vi "Opcode at X.vi"(9 "X Position":enum16{"First", "Second", "Third", "Fourth"}(ring), 11 "Opcode":u16 format="%04x") -> (2 "Opcode at X Position (U8)":u8 format="%02x")   [LabVIEW 2018]
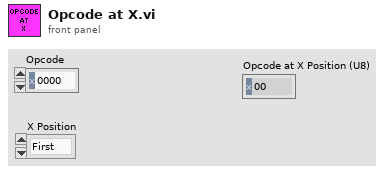
[diagram p1: front panel]
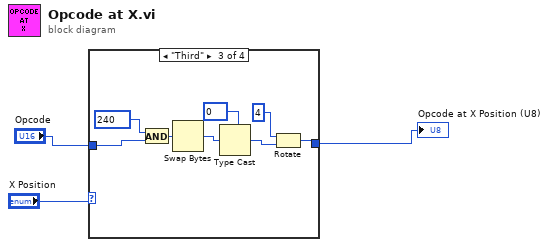
[diagram p0: block diagram]
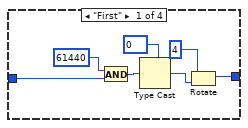
[diagram p2: hidden frame]
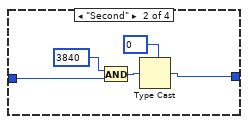
[diagram p3: hidden frame]
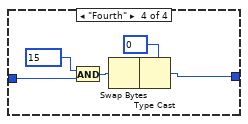
[diagram p4: hidden frame]
diagram:
  n1 = case shown="\"Third\"" "X Position" {
    tunnel: "Opcode" -> [w7 w12 w20 w26]
    tunnel: [w6 w11 w18 w25] -> w1
    frame "First" {
      n2 = And(x=u16 61440 ("y"), y=w7) -> (x .and. y?=w9:u16)
      n3 = Type Cast(type=u8 0, x=w9) -> (*(type *) &x=w5:u8)
      n4 = Rotate(1:w5, 2:u8 4 ("x")) -> (0:w6:u8)
    }
    frame "Second" {
      n5 = And(x=u16 3840 ("y"), y=w12) -> (x .and. y?=w14:u16)
      n6 = Type Cast(type=u8 0, x=w14) -> (*(type *) &x=w11:u8)
    }
    frame "Third" {
      n7 = And(x=u16 240 ("y"), y=w20) -> (x .and. y?=w22:u16)
      n8 = Swap Bytes(anything=w22) -> (byte swapped=w19:u16)
      n9 = Type Cast(type=u8 0, x=w19) -> (*(type *) &x=w16:u8)
      n10 = Rotate(1:w16, 2:i16 4 ("y")) -> (0:w18:u8)
    }
    frame "Fourth" {
      n11 = And(x=u16 15 ("y"), y=w26) -> (x .and. y?=w28:u16)
      n12 = Swap Bytes(anything=w28) -> (byte swapped=w24:u16)
      n13 = Type Cast(type=u8 0, x=w24) -> (*(type *) &x=w25:u8)
    }
  }
  "Opcode at X Position (U8)" <- w1
